vi "Check Sweep Complete.vi"(8 "Error In (no error)":errorcluster, 10 "Mode (T: Wait for sweep complete)":bool=TRUE, 11 "VISA Resource Name":refnum<visa-resource-name>) -> (0 "Error Out":errorcluster, 2 "Sweep Complete":bool, 3 "VISA Resource Name Out":refnum<visa-resource-name>)   [LabVIEW 2018, in "Agilent PNA Series.lvlib"]
doc: "This VI checks that the sweep is complete."
uses:
  Agilent PNA Series.lvlib
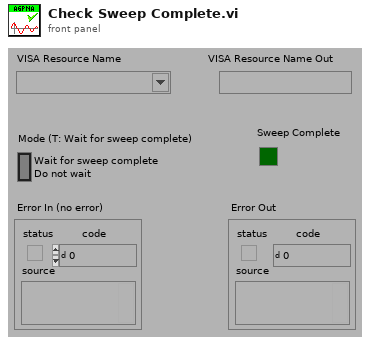
[diagram p1: front panel]
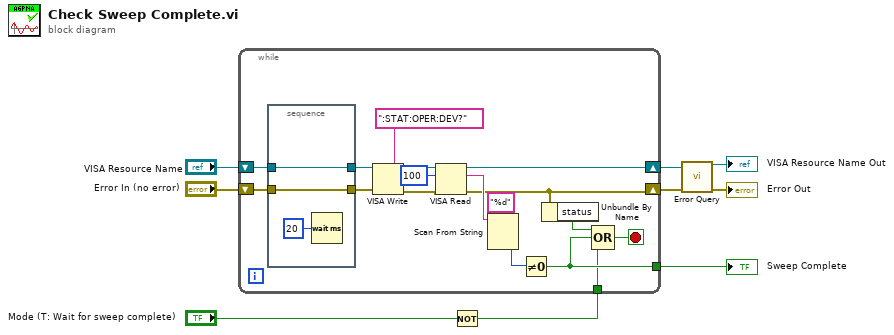
[diagram p0: block diagram]
diagram:
  n1 = Not(x="Mode (T: Wait for sweep complete)") -> (.not. x?=w5:bool)
  n2 = while {
    tunnel: w5 -> [w14]
    tunnel: [w15] -> w9
    shift-left: "Error In (no error)" -> [w11]
    shift-right: [w18] -> w3
    shift-left: "VISA Resource Name" -> [w13]
    shift-right: [w24] -> w4
    stop <- w16 stop-if-true
    n3 = stacked-sequence {
      tunnel: [w29] -> w12
      tunnel: w13 -> [w29]
      tunnel: [w28] -> w10
      tunnel: w11 -> [w28]
      frame #0 {
        n4 = Wait (ms)(milliseconds to wait=u32 20) -> ()  [unwired: 1 out]
      }
    }
    n5 = VISA Write(VISA resource name=w12, write buffer=":STAT:OPER:DEV?" ("write buffer (\"\")"), error in (no error)=w10) -> (VISA resource name out=w25:refnum<visa-resource-name>, error out=w23:errorcluster)  [unwired: 1 out]
    n6 = VISA Read(VISA resource name=w25, byte count=u32 100 ("byte count (0)"), error in (no error)=w23) -> (VISA resource name out=w24:refnum<visa-resource-name>, read buffer=w21:string, error out=w18:errorcluster)  [unwired: 1 out]
    n7 = Scan From String(format string="%d", input string=w21) -> (output 1=w19:i32)  [unwired: 3 in, 3 out]
    n8 = Not Equal To 0?(x=w19) -> (x != 0?=w15:bool)
    n9 = Unbundle By Name(w18) -> ("status"=w17:bool)
    n10 = Compound Arithmetic op=OR(w17, w15, w14) -> (w16:bool)
  }
  "Sweep Complete" <- w9
  n11 = call "Error Query.vi"("VISA Resource Name"=w4, "error in (no error)"=w3) -> ("VISA Resource Name Out"=→"VISA Resource Name Out":refnum<visa-resource-name>, "error out"=→"Error Out":errorcluster)  [unwired: 10 in, 2 out]
